vi "Get Measurement Library.vi"(8 "error in (no error)":errorcluster, 10 "Measurement Service Name":string, 11 "Project in":refnum<vi>) -> (0 "error out":errorcluster, 2 "Measurement Library Item":refnum<vi>)   [LabVIEW 2020, in "MeasurementService Editor.lvlib"]
uses:
  MeasurementService Editor.lvlib
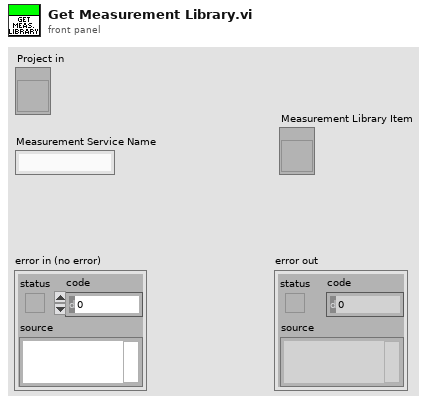
[diagram p1: front panel]
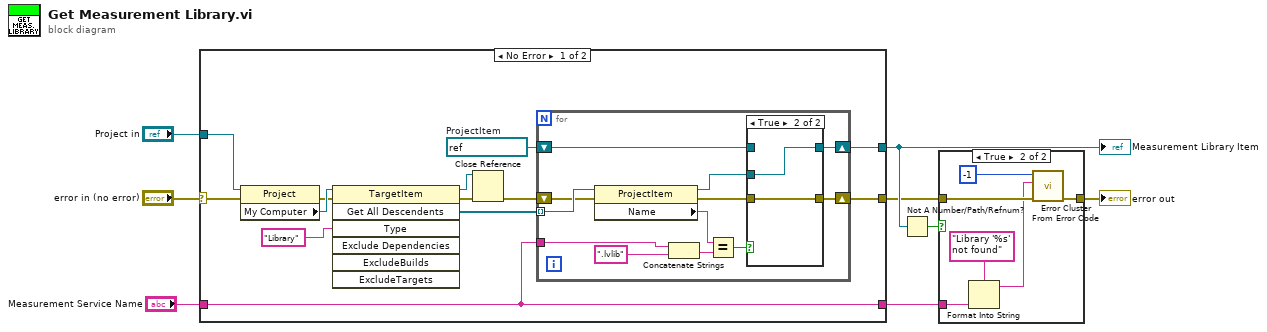
[diagram p0: block diagram]
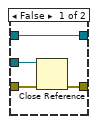
[diagram p3: hidden frame]
diagram:
  n1 = case shown="No Error" "error in (no error)" {
    selector: "error in (no error)" -> [w17 w41]
    tunnel: "Project in" -> [w21 _]
    tunnel: "Measurement Service Name" -> [w9 w40]
    tunnel: [w16 w41] -> w2
    tunnel: [w11 _] -> w5
    tunnel: [w9 w40] -> w1
    frame No Error {
      w12 = refnum<vi> refnum  # ProjectItem
      n2 = property class="Project"(reference=w21, error in=w17) -> (error out=w19:errorcluster, "My Computer"=w20:refnum<vi>)  [unwired: 1 out]
      n3 = invoke class="TargetItem" method="Get All Descendents"(reference=w20, error in=w19, "Type"="Library") -> (reference out=w14:refnum<vi>, error out=w15:errorcluster, "All Descendents"=w18:refnum<vi>[])  [unwired: 4 in, 4 out]
      n4 = Close Reference(reference=w14, error in (no error)=w15) -> (error out=w13:errorcluster)
      n5 = for {
        tunnel: w18 -> [w33] mode=indexing
        tunnel: w9 -> [w32]
        shift-right: [w24] -> w16
        shift-left: w13 -> [w28]
        shift-right: [w23] -> w11
        shift-left: w12 -> [w22]
        n6 = property class="ProjectItem"(reference=w33, error in=w28) -> (reference out=w26:refnum<vi>, error out=w27:errorcluster, "Name"=w30:string)
        n7 = Concatenate Strings(w32, ".lvlib" ("string")) -> (w29:string)
        n8 = Equal?(x=w30, y=w29) -> (x = y?=w25:bool)
        n9 = case shown="True" w25 {
          tunnel: w27 -> [w37 w39]
          tunnel: w26 -> [w34 w38]
          tunnel: [w36 w39] -> w24
          tunnel: [w35 w38] -> w23
          tunnel: w22 -> [w35 _]
          frame False {
            n10 = Close Reference(reference=w34, error in (no error)=w37) -> (error out=w36:errorcluster)
          }
          frame True {
          }
        }
      }
    }
    frame Error {
    }
  }
  "Measurement Library Item" <- w5
  n11 = Not A Number/Path/Refnum?(number/path/refnum=w5) -> (NaN/Path/Refnum?=w4:bool)
  n12 = case shown="True" w4 {
    tunnel: [w42 w48] -> w3
    tunnel: w2 -> [w42 w47]
    tunnel: w1 -> [_ w43]
    frame False {
    }
    frame True {
      n13 = Format Into String(format string="Library '%s' not found" ("initial string"), w43) -> (resulting string=w44:string)  [unwired: 2 in, 1 out]
      n14 = call <vilib>:"Error Cluster From Error Code.vi"("error in (no error)"=w47, "error message (\"\")"=w44, "error code (0)"=-1) -> ("error out"=w48:errorcluster)  [unwired: 6 in]
    }
  }
  "error out" <- w3
